vi "MoveCamera.vi"(8 "error in (no error)":errorcluster, 11 "Game in":refnum<class "Game.lvclass">) -> (0 "error out":errorcluster, 3 "Game out":refnum<class "Game.lvclass">)   [LabVIEW 2019, in "RT_Game.lvlib" / "Game.lvclass"]
uses:
  Game.lvclass
  Coordinate.ctl
  Game.lvclass/Game.ctl
  Globals.vi
  <vilib>/Utility/error.llb/Error Cluster From Error Code.vi
  <vilib>/rvi/errors/niLvFpgaAdjustHostInterfaceError.vi
  <vilib>/rvi/interface/nirviReadWriteControl/nirviReadWriteControl.xnode
  FPGA_Interface.ctl
  FPGA Bitfiles/myriogameconsole_FPGATarget_Main_ntsPRcBZGxk.lvbitx
  RT_Game.lvlib
  NiFpgaLv.dll
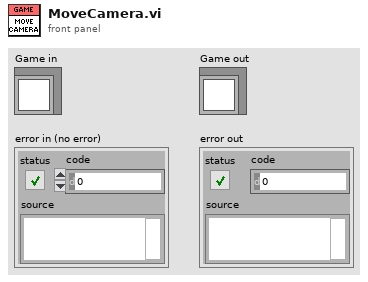
[diagram p1: front panel]
types:
  T1 = typedef "RT_Game.lvlib/Game.lvclass/Coordinate.ctl" = cluster{"x":dbl, "y":dbl}
  T2 = typedef "FPGA_Interface.ctl" = refnum<k20>
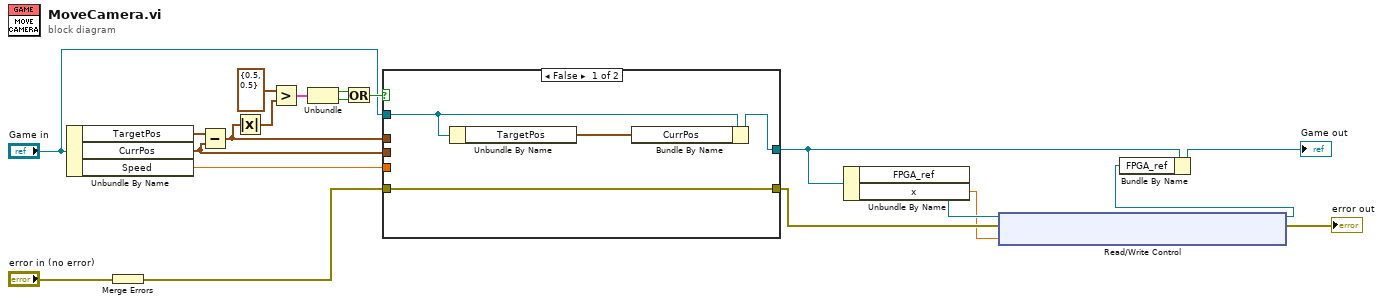
[diagram p0: block diagram]
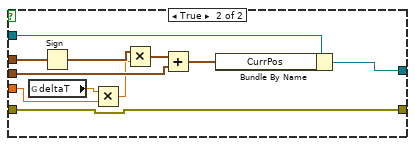
[diagram p2: hidden frame]
diagram:
  n1 = Unbundle By Name("Game in") -> ("TargetPos"=w11:T1, "CurrPos"=w13:T1, "Speed"=w12:dbl)
  n2 = Merge Errors("error in (no error)") -> (w8:errorcluster)
  n3 = Subtract(x=w11, y=w13) -> (x-y=w14:T1)
  n4 = Absolute Value(x=w14) -> (abs(x)=w20:T1)
  n5 = Greater?(x=T1 {"x"=0.5, "y"=0.5}, y=w20) -> (0:w16:cluster{"x":bool, "y":bool})
  n6 = Unbundle(w16) -> ("x"=w17:bool, "y"=w18:bool)
  n7 = Or(x=w17, y=w18) -> (x .or. y?=w19:bool)
  n8 = case shown="False" w19 {
    tunnel: "Game in" -> [w23 w35]
    tunnel: [w22 w34] -> w5
    tunnel: w12 -> [_ w32]
    tunnel: w13 -> [_ w31]
    tunnel: w14 -> [_ w29]
    tunnel: w8 -> [w24 w25]
    tunnel: [w24 w25] -> w7
    frame False {
      n9 = Unbundle By Name(w23) -> ("TargetPos"=w21:T1)
      n10 = Bundle By Name(cluster=w23, "CurrPos"=w21) -> (w22:refnum<class "Game.lvclass">)
    }
    frame True {
      n11 = global read "Globals.vi" "deltaT"() -> (w27:dbl)
      n12 = Sign(1:w29) -> (0:w33:T1)
      n13 = Multiply(x=w27, y=w32) -> (x*y=w28:dbl)
      n14 = Multiply(x=w33, y=w28) -> (x*y=w26:T1)
      n15 = Add(x=w26, y=w31) -> (x+y=w30:T1)
      n16 = Bundle By Name(cluster=w35, "CurrPos"=w30) -> (w34:refnum<class "Game.lvclass">)
    }
  }
  n17 = Unbundle By Name(w5) -> ("FPGA_ref"=w3:T2, "x"=w1:dbl)
  n18 = xnode "Read/Write Control"("FPGA VI Reference In"=w3, "error in"=w7, "x_Shift"=w1) -> ("FPGA VI Reference Out"=w2:T2, "error out"=→"error out":errorcluster)
  n19 = Bundle By Name(cluster=w5, "FPGA_ref"=w2) -> (→"Game out":refnum<class "Game.lvclass">)
